vi "Format Into Banking Table.vi"(8 "error in (no error)":errorcluster, 11 "Banking Statement.lvclass":refnum<class "Banking Statement.lvclass">) -> (0 "error out":errorcluster, 3 "Table Row":string[][](array[string]))   [LabVIEW 2018, in "Banking Statement.lvclass"]
uses:
  Banking Statement.lvclass
  C:/GitRepos/Filthy-Lucre-Budgetizer/source/support/classes/Statement/Statement.lvclass
  Transaction/Transaction.lvclass
  Statement/Statement.lvclass
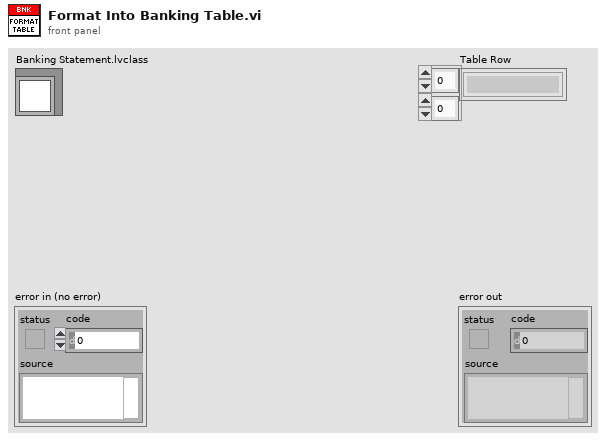
[diagram p1: front panel]
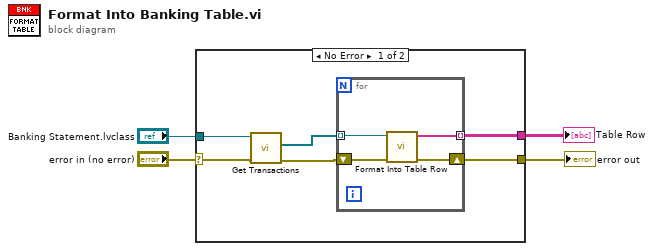
[diagram p0: block diagram]
diagram:
  n1 = case shown="No Error" "error in (no error)" {
    selector: "error in (no error)" -> [w7 w15]
    tunnel: [w10 w15] -> w3
    tunnel: "Banking Statement.lvclass" -> [w8 _]
    tunnel: [w9 _] -> w1
    frame No Error {
      n2 = call "Get Transactions.vi"("error in (no error)"=w7, "Statement in"=w8) -> ("error out"=w6:errorcluster, "Transactions"=w5:refnum<class "Transaction.lvclass">[])  [unwired: 7 in, 1 out]
      n3 = for {
        tunnel: w5 -> [w14] mode=indexing
        tunnel: [w13] -> w9 mode=indexing
        shift-right: [w11] -> w10
        shift-left: w6 -> [w12]
        n4 = call "Format Into Table Row.vi"("error in (no error)"=w12, "Transaction in"=w14) -> ("error out"=w11:errorcluster, "Table Row"=w13:string[])  [unwired: 8 in]
      }
    }
    frame Error {
    }
  }
  "error out" <- w3
  "Table Row" <- w1
